vi "channel specification from user VI path.vi"(8 "error in (no error)":errorcluster, 11 "User VI Path in":path) -> (0 "error out":errorcluster, 3 "Channel Specification out":T1[](array[typedef]))   [LabVIEW 2013]
uses:
  channel configuration.ctl
  <vilib>/NI/Tag Bus Module Framework/channel/channel classification.ctl
  <vilib>/NI/Tag Bus/tag/Data Type.ctl
  <vilib>/NI/Tag Bus/tag/tag descriptor.lvclass
  <vilib>/NI/Tag Bus Module Framework/channel/TBM channel.lvclass
  FixedChannelTBModuleDecideFeatures.lvclass
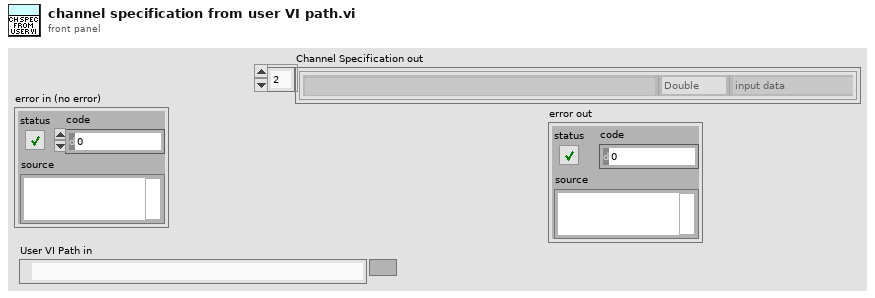
[diagram p1: front panel]
types:
  T1 = typedef "FixedChannelTBModuleDecideFeatures.lvclass/channel configuration.ctl" = cluster{"Name":string, "channel classification":T2, "data type":T3}
  T2 = typedef "TBM channel.lvclass/channel classification.ctl" = enum16{"input data", "output data", "processing parameter", "processing result"}
  T3 = typedef "tag bus.lvlib/tag descriptor.lvclass/Data Type.ctl" = enum16{"Double", "Single", "I64", "I32", "I16", "I8", "U64", "U32", "U16", "U8", "Boolean", "String", "Array of Double", "Array of Single", "Array of I64", "Array of I32", "Array of I16", "Array of I8", "Array of U64", "Array of U32", "Array of U16", "Array of U8", "Array of Boolean", "Array of String"}
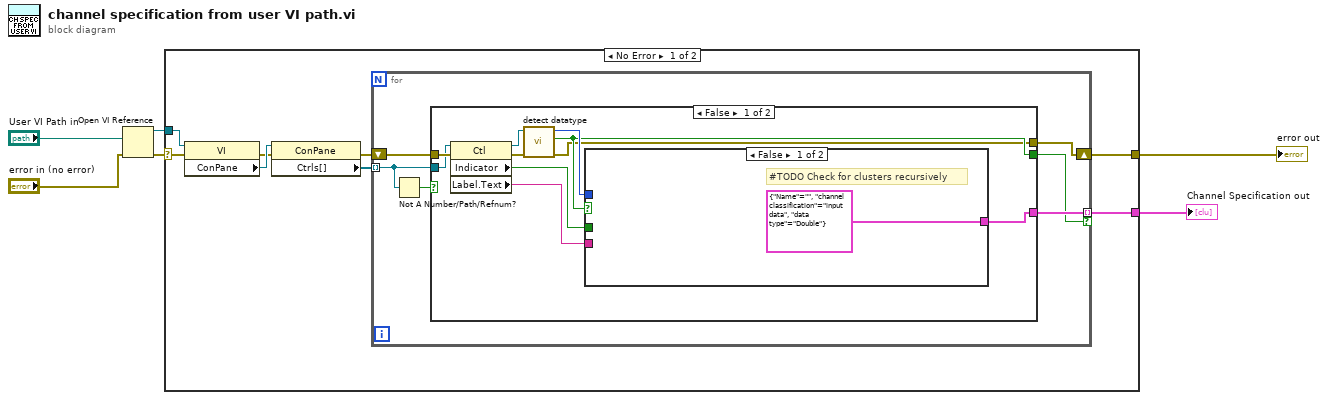
[diagram p0: block diagram]
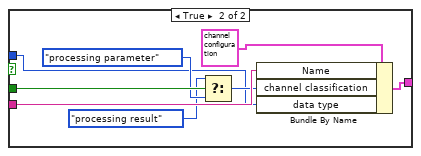
[diagram p2: hidden frame]
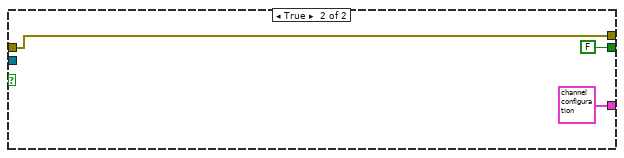
[diagram p3: hidden frame]
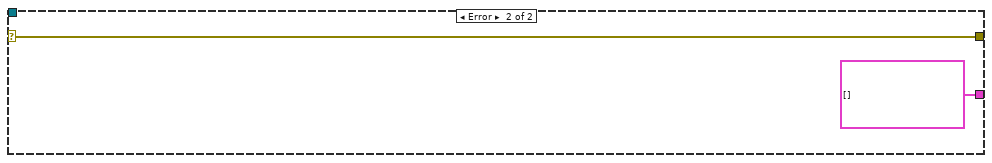
[diagram p4: hidden frame]
diagram:
  n1 = Open VI Reference(vi path="User VI Path in", error in (no error)="error in (no error)") -> (vi reference=w2:refnum<vi>, error out=w5:errorcluster)  [unwired: 4 in]
  n2 = case shown="No Error" w5 {
    selector: w5 -> [w12 w44]
    tunnel: [w8 w44] -> w3
    tunnel: w2 -> [w14 _]
    tunnel: [w7 T1[] []] -> w1
    frame No Error {
      n3 = property class="VI"(reference=w14, error in=w12) -> (error out=w11:errorcluster, "ConPane"=w13:refnum<vi>)  [unwired: 1 out]
      n4 = property class="ConPane"(reference=w13, error in=w11) -> (error out=w9:errorcluster, "Ctrls[]"=w10:refnum<vi>[])  [unwired: 1 out]
      n5 = for {
        tunnel: w10 -> [w16] mode=indexing
        shift-right: [w18] -> w8
        shift-left: w9 -> [w17]
        tunnel: [w20] -> w7 mode=indexing if=w19
        n6 = Not A Number/Path/Refnum?(number/path/refnum=w16) -> (NaN/Path/Refnum?=w15:bool)
        n7 = case shown="False" w15 {
          tunnel: [w28 T1 {"Name"="", "channel classification"=enum."input data", "data type"=enum."Double"} ("Channel Configuration")] -> w20
          tunnel: [w26 FALSE ("is supported?")] -> w19
          tunnel: [w24 w41] -> w18
          tunnel: w17 -> [w23 w41]
          tunnel: w16 -> [w21 _]
          frame False {
            n8 = property class="Ctl"(reference=w21, error in=w23) -> (reference out=w22:refnum<vi>, error out=w25:errorcluster, "Indicator"=w29:bool, "Label.Text"=w30:string)
            n9 = call "detect datatype.vi"("error in (no error)"=w25, "Ctl Refnum"=w22) -> ("error out"=w24:errorcluster, "is supported?"=w26:bool, "data type"=w27:T3)  [unwired: 6 in]
            n10 = case shown="False" w26 {
              tunnel: w30 -> [_ w39]
              tunnel: w29 -> [_ w37]
              tunnel: [T1 {"Name"="", "channel classification"=enum."input data", "data type"=enum."Double"} ("Channel Configuration") w33] -> w28
              tunnel: w27 -> [_ w32]
              frame False {
                # "#TODO Check for clusters recursively"
              }
              frame True {
                n11 = Select(t=channel_classification."processing result", s=w37, f=channel_classification."processing parameter" ("channel classification")) -> (s? t:f=w36:T2)
                n12 = Bundle By Name(cluster=T1 {"Name"="", "channel classification"=enum."input data", "data type"=enum."Double"} ("Channel Configuration"), "Name"=w39, "channel classification"=w36, "data type"=w32) -> (w33:T1)
              }
            }
          }
          frame True {
          }
        }
      }
    }
    frame Error {
    }
  }
  "Channel Specification out" <- w1
  "error out" <- w3
